vi "Test VI.vi"() -> ()   [LabVIEW 2014]
panel:
  out "Boolean":bool
  in  "Temp Control":dbl(knob) scale=0.0..100.0
  out "Thermometer":dbl(slide) scale=0.0..100.0
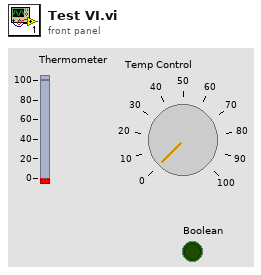
[diagram p1: front panel]
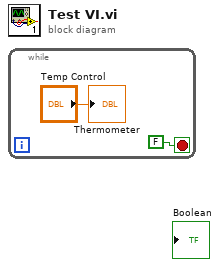
[diagram p0: block diagram]
diagram:
  n1 = while {
    stop <- FALSE stop-if-true
    "Thermometer" <- "Temp Control"
  }
